vi "Image control reference.vi"() -> ()   [LabVIEW 2017]
panel:
  in  "Image control":refnum<vi>
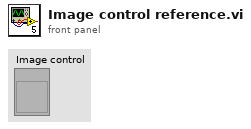
[diagram p1: front panel]
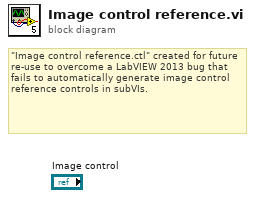
[diagram p0: block diagram]
diagram:
  # "\"Image control reference.ctl\" created for future re-use to overcome a LabVIEW 2013 bug that fails to automatically generate image control reference controls in subVIs."
